vi "CloseAllTasks.vi"(0 "Task Array":refnum<k21>[](array[refnum]), 3 "error in (no error)":errorcluster) -> (10 "error out":errorcluster)   [LabVIEW 2016]
doc: "Close out all tasks input in task array"
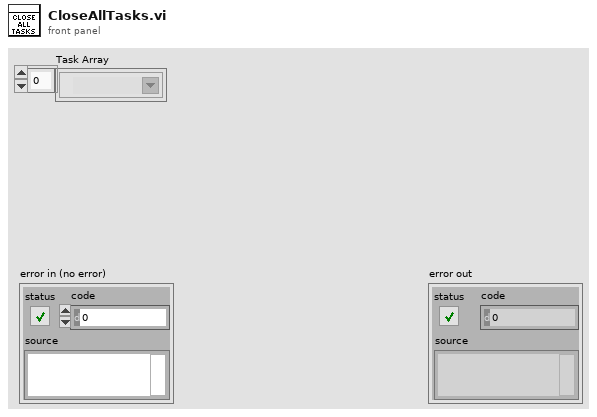
[diagram p1: front panel]
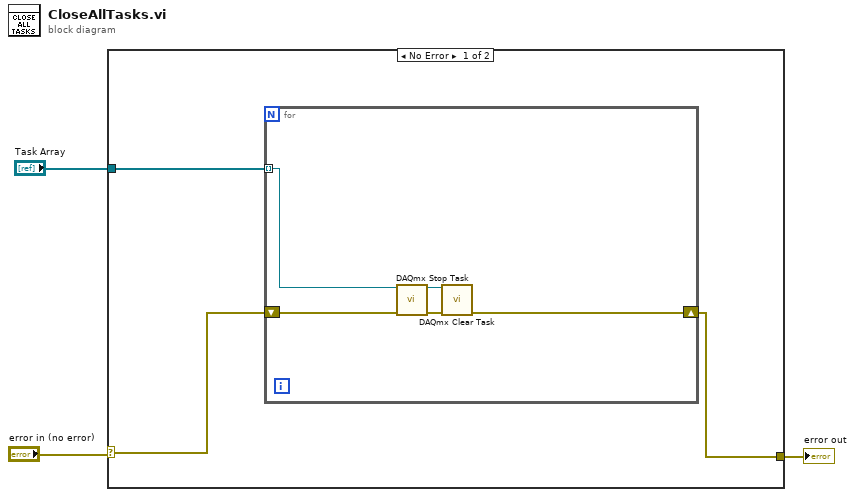
[diagram p0: block diagram]
diagram:
  n1 = case shown="No Error" "error in (no error)" {
    selector: "error in (no error)" -> [w5 w12]
    tunnel: "Task Array" -> [w6 _]
    tunnel: [w4 w12] -> w1
    frame No Error {
      n2 = for {
        tunnel: w6 -> [w8] mode=indexing
        shift-right: [w9] -> w4
        shift-left: w5 -> [w10]
        n3 = call <vilib>:"DAQmx Stop Task.vi"("task/channels in"=w8, "error in"=w10) -> ("task out"=w7:refnum<k21>, "error out"=w11:errorcluster)  [unwired: 12 in]
        n4 = call <vilib>:"DAQmx Clear Task.vi"("task in"=w7, "error in"=w11) -> ("error out"=w9:errorcluster)  [unwired: 13 in]
      }
    }
    frame Error {
    }
  }
  "error out" <- w1
